vi "Separate 4ROI.vi"(6 "SearchArea(0.3)":dbl=0.3 format="%#_13g", 7 "ROI Descriptor":T2 {"Contours"."Type" items=["No Selection", "Point", "Line", "Rectangle", "Oval", "Polygon", "Freehand Region", "Annulus", "Unused2", "Unused3", "Broken Line", "Freehand Line", "Rotated Rectangle"]}) -> (0 "Bottom ROI":T1 {"Contours"."Type" items=["No Selection", "Point", "Line", "Rectangle", "Oval", "Polygon", "Free", "Annulus", "Unused2", "Unused3", "Broken Line", "Free Hand Line", "Rotated Rectangle"]}, 1 "Right ROI":T1 {"Contours"."Type" items=["No Selection", "Point", "Line", "Rectangle", "Oval", "Polygon", "Free", "Annulus", "Unused2", "Unused3", "Broken Line", "Free Hand Line", "Rotated Rectangle"]}, 2 "Top ROI":T1 {"Contours"."Type" items=["No Selection", "Point", "Line", "Rectangle", "Oval", "Polygon", "Free", "Annulus", "Unused2", "Unused3", "Broken Line", "Free Hand Line", "Rotated Rectangle"]}, 3 "Left ROI":T1 {"Contours"."Type" items=["Separate 4ROI.viNo Selection", "Point", "Line", "Rectangle", "Oval", "Polygon", "Free", "Annulus", "Unused2", "Unused3", "Broken Line", "Free Hand Line", "Rotated Rectangle"]})   [LabVIEW 2015]
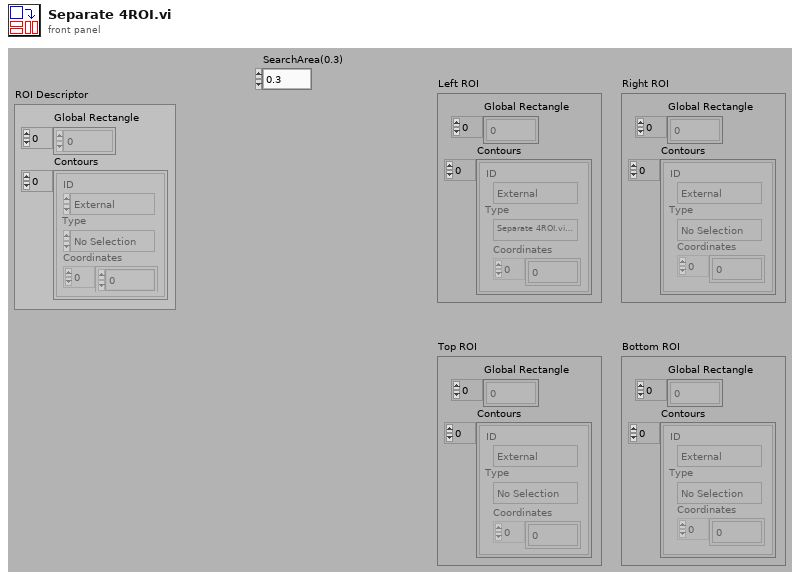
[diagram p1: front panel]
types:
  T1 = cluster{"Global Rectangle":i32[], "Contours":cluster{"ID":enum32{"External", "Internal"}, "Type":u32, "Coordinates":i32[]}[]}
  T2 = typedef "ROI Descriptor" = cluster{"Global Rectangle":i32[], "Contours":cluster{"ID":enum32{"External", "Internal"}, "Type":u32, "Coordinates":i32[]}[]}
  T3 = cluster{"ID":enum32{"External", "Internal"}, "Type":u32, "Coordinates":i32[]}[]
  T4 = cluster{"ID":enum32{"External", "Internal"}, "Type":u32, "Coordinates":i32[]}
  T5 = enum32{"No Selection", "Point", "Line", "Rectangle", "Oval", "Polygon", "Free", "Unused1", "Unused2", "Unused3", "Broken Line", "Free Hand Line"}
  T6 = cluster{"ID":enum32{"External", "Internal"}, "Type":enum32{"No Selection", "Point", "Line", "Rectangle", "Oval", "Polygon", "Free", "Unused1", "Unused2", "Unused3", "Broken Line", "Free Hand Line"}, dbl[]}
  T7 = cluster{"ID":enum32{"External", "Internal"}, "Type":enum32{"No Selection", "Point", "Line", "Rectangle", "Oval", "Polygon", "Free", "Unused1", "Unused2", "Unused3", "Broken Line", "Free Hand Line"}, dbl[]}[]
  T8 = cluster{"Global Rectangle":i32[], cluster{"ID":enum32{"External", "Internal"}, "Type":enum32{"No Selection", "Point", "Line", "Rectangle", "Oval", "Polygon", "Free", "Unused1", "Unused2", "Unused3", "Broken Line", "Free Hand Line"}, dbl[]}[]}
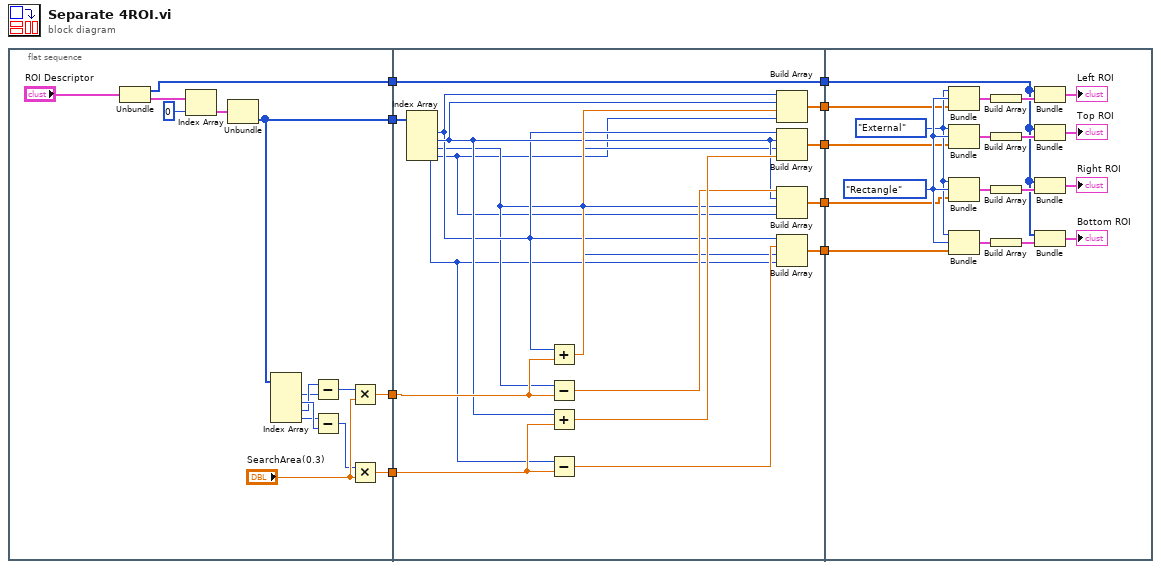
[diagram p0: block diagram]
diagram:
  n1 = flat-sequence {
    tunnel: [w21] -> w9
    tunnel: [w12] -> w8
    tunnel: [w11] -> w2
    tunnel: [w10] -> w1
    tunnel: w9 -> [w38]
    tunnel: w8 -> [w39]
    tunnel: [w38] -> w7
    tunnel: [w37] -> w6
    tunnel: [w36] -> w5
    tunnel: [w35] -> w4
    tunnel: [w34] -> w3
    tunnel: w2 -> [w33]
    tunnel: w1 -> [w32]
    tunnel: w7 -> [w45]
    tunnel: w6 -> [w44]
    tunnel: w5 -> [w43]
    tunnel: w4 -> [w42]
    tunnel: w3 -> [w41]
    frame #0 {
      n2 = Unbundle("ROI Descriptor") -> ("Global Rectangle"=w21:i32[], "Contours"=w22:T3)
      n3 = Index Array(array=w22, index=0 ("Index")) -> (element=w24:T4)
      n4 = Unbundle(w24) -> ("Coordinates"=w12:i32[])  [unwired: 2 out]
      n5 = Index Array(array=w12) -> (element #1=w13:i32, element #2=w16:i32, element #3=w14:i32, element #4=w15:i32)  [unwired: 4 in]
      n6 = Subtract(x=w14, y=w13) -> (x-y=w17:i32)
      n7 = Subtract(x=w15, y=w16) -> (x-y=w18:i32)
      n8 = Multiply(x=w17, y="SearchArea(0.3)") -> (x*y=w10:dbl)
      n9 = Multiply(x=w18, y="SearchArea(0.3)") -> (x*y=w11:dbl)
    }
    frame #1 {
      n10 = Index Array(array=w39) -> (element #1=w28:i32, element #2=w29:i32, element #3=w26:i32, element #4=w25:i32)  [unwired: 4 in]
      n11 = Add(x=w28, y=w32) -> (x+y=w40:dbl)
      n12 = Subtract(x=w26, y=w32) -> (x-y=w30:dbl)
      n13 = Add(x=w29, y=w33) -> (x+y=w31:dbl)
      n14 = Subtract(x=w25, y=w33) -> (x-y=w27:dbl)
      n15 = Build Array(w28, w29, w40, w25) -> (w37:dbl[])
      n16 = Build Array(w28, w29, w26, w31) -> (w36:dbl[])
      n17 = Build Array(w30, w29, w26, w25) -> (w35:dbl[])
      n18 = Build Array(w28, w27, w26, w25) -> (w34:dbl[])
    }
    frame #2 {
      w59 = T5."Rectangle" ("Type")
      w58 = enum32{"External", "Internal"}."External" ("ID")
      n19 = Bundle("ID"=w58, "Type"=w59, w44) -> (w48:T6)  [unwired: 1 out]
      n20 = Bundle("ID"=w58, "Type"=w59, w43) -> (w53:T6)  [unwired: 1 out]
      n21 = Bundle("ID"=w58, "Type"=w59, w42) -> (w49:T6)  [unwired: 1 out]
      n22 = Bundle("ID"=w58, "Type"=w59, w41) -> (w52:T6)  [unwired: 1 out]
      n23 = Build Array(w48) -> (w46:T7)
      n24 = Build Array(w53) -> (w54:T7)
      n25 = Build Array(w49) -> (w47:T7)
      n26 = Build Array(w52) -> (w55:T7)
      n27 = Bundle("Global Rectangle"=w45, w46) -> (→"Left ROI":T8)  [unwired: 1 out]
      n28 = Bundle("Global Rectangle"=w45, w54) -> (→"Top ROI":T8)  [unwired: 1 out]
      n29 = Bundle("Global Rectangle"=w45, w47) -> (→"Right ROI":T8)  [unwired: 1 out]
      n30 = Bundle("Global Rectangle"=w45, w55) -> (→"Bottom ROI":T8)  [unwired: 1 out]
    }
  }
